vi "scan.vi"(8 "error in (no error)":errorcluster, 11 "Input":string="34,45,89") -> (0 "error out":errorcluster, 3 "Output":string)   [LabVIEW 2014]
uses:
  <userlib>/Nanonis Prog Interface V5/Nanonis Prog Interface.lvlib
panel:
  in  "Channel":u8(ring)=14 items=["Current"=0, "Z (m)"=14]
  in  "Direction: Fwd/Bwd (T=Fwd)":bool=TRUE
  in  "milliseconds to wait":u32=3000
  in  "Angle (deg)":sgl=nan caption="Angle (deg) (NaN=no change)" format="%.2f"
  in  "Size (m)":cluster{"Width":sgl, "Height":sgl}={"Width"=1e-08, "Height"=1e-08} caption="Size (m) (NaN=no change)" {"Height" format="%.2p"; "Width" format="%.2p"}
  out "size(s)":i32=3
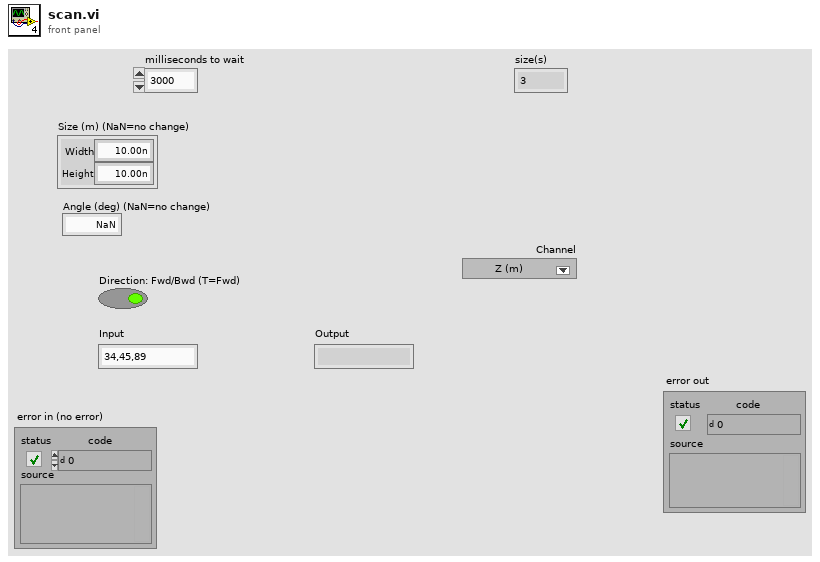
[diagram p1: front panel]
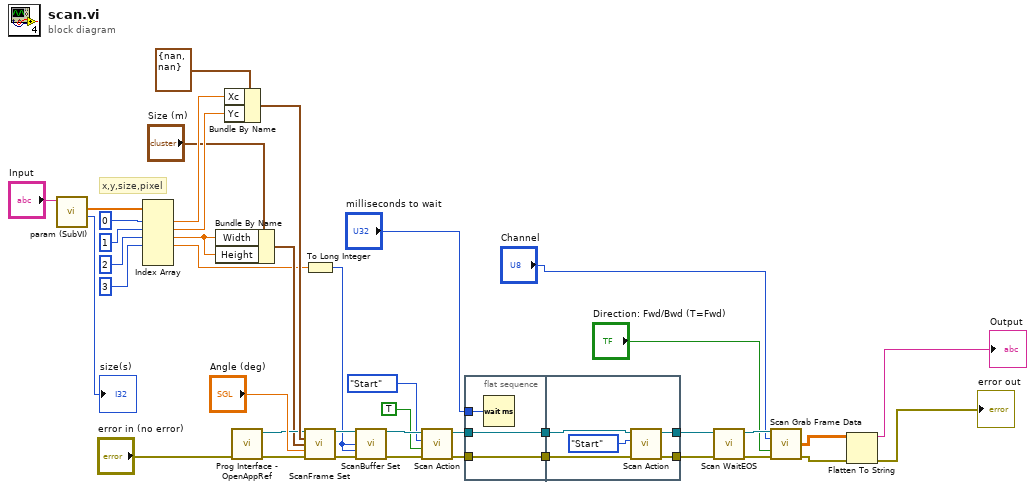
[diagram p0: block diagram]
diagram:
  # "x,y,size,pixel"
  n1 = call <userlib>:"param (SubVI).vi"("Input"="Input") -> ("num"=→"size(s)":i32, "parm"=w39:dbl[])  [unwired: 8 in, 1 out]
  n2 = Index Array(array=w39, index #1=0 ("index"), index #2=1 ("index"), index #3=2 ("index"), index #4=3 ("index")) -> (element #1=w37:dbl, element #2=w36:dbl, element #3=w9:dbl, element #4=w7:dbl)  [unwired: 2 in, 2 out]
  n3 = Bundle By Name(cluster="Size (m)", "Width"=w9, "Height"=w9) -> (w8:cluster{"Width":sgl, "Height":sgl})
  n4 = Bundle By Name(cluster=cluster{"Xc":sgl, "Yc":sgl} {"Xc"=nan, "Yc"=nan} ("Center coordinates (m)"), "Xc"=w37, "Yc"=w36) -> (w35:cluster{"Xc":sgl, "Yc":sgl})
  n5 = call <userlib>:"Prog Interface - OpenAppRef.vi"("Error in (no error)"="error in (no error)") -> ("Error out"=w21:errorcluster, "Application reference"=w22:refnum<vi>)  [unwired: 5 in]
  n6 = To Long Integer(number=w7) -> (32bit integer=w6:i32)
  n7 = call <userlib>:"ScanFrame Set.vi"("Application ref in"=w22, "Center coordinates (m)"=w35, "Size (m)"=w8, "Angle (deg)"="Angle (deg)", "error in (no error)"=w21) -> ("Application ref out"=w33:refnum<vi>, "error out"=w32:errorcluster)  [unwired: 9 in]
  n8 = call <userlib>:"ScanBuffer Set.vi"("Application ref in"=w33, "Pixels"=w6, "Lines"=w6, "error in (no error)"=w32) -> ("Application ref out"=w30:refnum<vi>, "error out"=w31:errorcluster)  [unwired: 10 in]
  n9 = call <userlib>:"Scan Action.vi"("error in (no error)"=w31, "Direction: up/down (T=up)"=TRUE, "Scan action (Start)"=enum16{"Start", "Stop", "Pause", "Resume"}."Start", "Application ref in"=w30) -> ("error out"=w26:errorcluster, "Application ref out"=w27:refnum<vi>)  [unwired: 5 in]
  n10 = flat-sequence {
    tunnel: w27 -> [w43]
    tunnel: w26 -> [w42]
    tunnel: "milliseconds to wait" -> [w44]
    tunnel: [w43] -> w24
    tunnel: [w42] -> w23
    tunnel: w24 -> [w49]
    tunnel: w23 -> [w48]
    tunnel: [w46] -> w19
    tunnel: [w45] -> w18
    frame #0 {
      n11 = Wait (ms)(milliseconds to wait=w44) -> ()  [unwired: 1 out]
    }
    frame #1 {
      n12 = call <userlib>:"Scan Action.vi"("error in (no error)"=w48, "Scan action (Start)"=enum16{"Start", "Stop", "Pause", "Resume"}."Start", "Application ref in"=w49) -> ("error out"=w45:errorcluster, "Application ref out"=w46:refnum<vi>)  [unwired: 6 in]
    }
  }
  n13 = call <userlib>:"Scan WaitEOS.vi"("error in (no error)"=w18, "Application ref in"=w19) -> ("error out"=w15:errorcluster, "Application ref out"=w17:refnum<vi>)  [unwired: 5 in, 2 out]
  n14 = call <userlib>:"Scan Grab Frame Data.vi"("Application ref in"=w17, "Channel index (0-23)"="Channel", "Direction: Fwd/Bwd (T=Fwd)"="Direction: Fwd/Bwd (T=Fwd)", "error in (no error)"=w15) -> ("Scan frame data"=w5:sgl[][], "error out"=w4:errorcluster)  [unwired: 7 in, 3 out]
  n15 = Flatten To String(anything=w5, error in (no error)=w4) -> (data string=→"Output":string, error out=→"error out":errorcluster)  [unwired: 2 in, 1 out]
